vi "SSC DCPower Configure Output Function.vi"(0 "DCPower SSC in":T2[](array[typedef]), 5 "Output Function":T1=1006 items=["DC Voltage"=1006, "DC Current"=1007, "Pulse Voltage"=1049, "Pulse Current"=1050], 11 "error in":errorcluster) -> (4 "DCPower SSC out":T2[](array[typedef]), 15 "error out":errorcluster)   [LabVIEW 2019]
doc: "This VI configures the output function of the instrument sessions. The tasks must be aborted when calling this method."
uses:
  SSC DCPower.ctl
  <instrlib>/niDCPower/nidcpower.llb/niDCPower Output Function.ctl
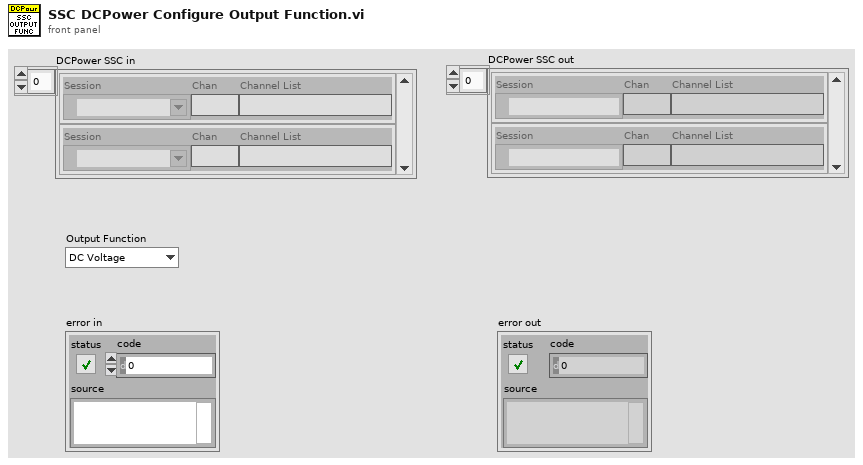
[diagram p1: front panel]
types:
  T1 = typedef "niDCPower Output Function.ctl" = i32
  T2 = typedef "SSC DCPower.ctl" = cluster{"Session":refnum<k15>, "Chan":string, "Channel List":string}
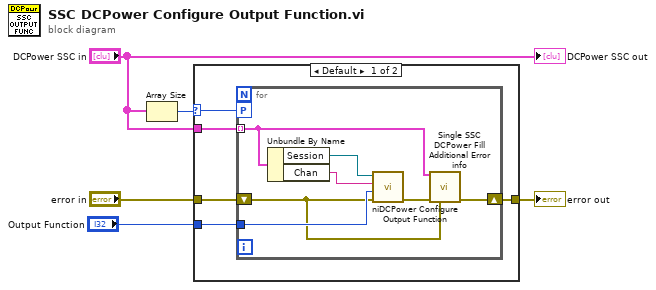
[diagram p0: block diagram]
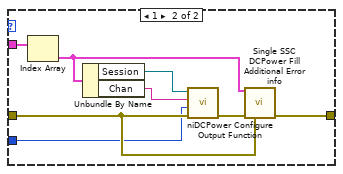
[diagram p2: hidden frame]
diagram:
  n1 = Array Size(array="DCPower SSC in") -> (size(s)=w3:i32)
  n2 = case shown="Default" w3 {
    selector: w3 -> [w8 _]
    tunnel: [w10 w25] -> w5
    tunnel: "error in" -> [w9 w24]
    tunnel: "DCPower SSC in" -> [w7 w23]
    tunnel: "Output Function" -> [w6 w22]
    frame Default {
      n3 = for {
        workers-P: w8 -> [_]
        tunnel: w7 -> [w12] mode=indexing
        shift-right: [w13] -> w10
        shift-left: w9 -> [w11]
        tunnel: w6 -> [w14]
        n4 = Unbundle By Name(w12) -> ("Session"=w17:refnum<k15>, "Chan"=w15:string)
        n5 = call <instrlib>:"niDCPower Configure Output Function.vi"("error in (no error)"=w11, "output function"=w14, "channel name"=w15, "instrument handle"=w17) -> ("error out"=w16:errorcluster)  [unwired: 6 in, 1 out]
        n6 = call "Single SSC DCPower Fill Additional Error info.vi"("DCPower SSC in"=w12, "error in"=w16, "previous error in"=w11) -> ("error out"=w13:errorcluster)  [unwired: 12 in]
      }
    }
    frame 1 {
      n7 = Index Array(array=w23) -> (element=w18:T2)  [unwired: 1 in]
      n8 = Unbundle By Name(w18) -> ("Session"=w21:refnum<k15>, "Chan"=w19:string)
      n9 = call <instrlib>:"niDCPower Configure Output Function.vi"("error in (no error)"=w24, "output function"=w22, "channel name"=w19, "instrument handle"=w21) -> ("error out"=w20:errorcluster)  [unwired: 6 in, 1 out]
      n10 = call "Single SSC DCPower Fill Additional Error info.vi"("DCPower SSC in"=w18, "error in"=w20, "previous error in"=w24) -> ("error out"=w25:errorcluster)  [unwired: 12 in]
    }
  }
  "error out" <- w5
  "DCPower SSC out" <- "DCPower SSC in"
